vi "DAQmx Create Channel (TEDS-AI-Pressure-Bridge).vi"(0 "task in":refnum<k21>, 1 "maximum value":dbl=100.0 format="%0.2f", 2 "minimum value":dbl=-100.0 format="%0.2f", 5 "physical channels":tag, 7 "name to assign":string, 9 "units":i32(ring)=15879 items=["Pascals"=10081, "psi"=15879, "bar"=15880, "From Custom Scale"=10065], 11 "error in":errorcluster, 12 "custom scale name":tag, 13 "voltage excitation source":i32(ring)=10200 items=["Internal"=10200, "External"=10167], 14 "voltage excitation value":dbl=2.5) -> (4 "task out":refnum<k21>, 15 "error out":errorcluster)   [LabVIEW 2020]
doc: "Creates channel(s) that use a Wheatstone bridge to measure pressure. You must configure the physical channel(s) with TEDS information to use this VI. NI-DAQmx scales electrical values to physical values according to that TEDS information."
uses:
  nilvaiu.dll
panel:
  # "input limits"
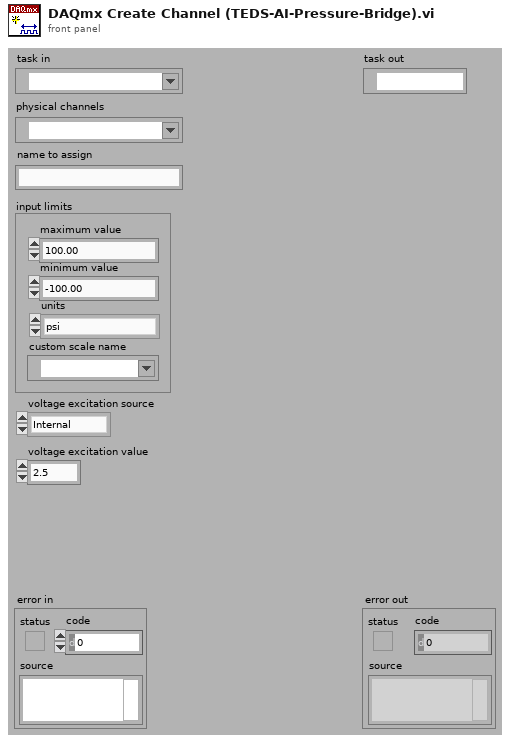
[diagram p1: front panel]
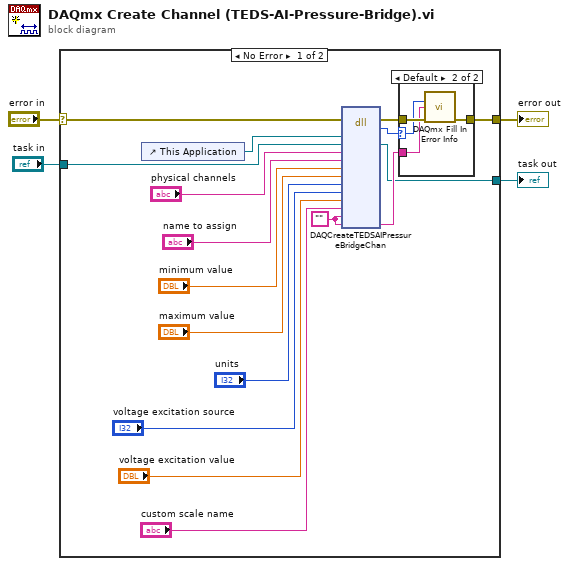
[diagram p0: block diagram]
diagram:
  n1 = case shown="No Error" "error in" {
    selector: "error in" -> [w11 w27]
    tunnel: [w18 w27] -> w4
    tunnel: "task in" -> [w14 w28]
    tunnel: [w17 w28] -> w1
    frame No Error {
      w5 = ""
      n2 = control-ref of="This Application"() -> (w16:refnum<vi>)
      n3 = dll-call lib="nilvaiu.*" fn="DAQCreateTEDSAIPressureBridgeChan"(error in=w11, "lvAppRef"=w16, "refObjPtr"=w14, "physicalChannelName"="physical channels", "channelNameIn"="name to assign", "minVal"="minimum value", "maxVal"="maximum value", "units"="units", "voltageExcitSource"="voltage excitation source", "voltageExcitVal"="voltage excitation value", "customScaleName"="custom scale name", "channelNamesOut"=w5, "extendedErrorInfo"=w5) -> (error out=w20:errorcluster, "return type"=w21:i32, "refObjPtr"=w17:refnum<k21>, "extendedErrorInfo"=w19:string)  [unwired: 12 in, 1 out]
      n4 = case shown="Default" w21 {
        selector: w21 -> [_ w24]
        tunnel: w20 -> [w22 w26]
        tunnel: [w22 w25] -> w18
        tunnel: w19 -> [_ w23]
        frame 0 {
        }
        frame Default {
          n5 = call "DAQmx Fill In Error Info.vi"("status code"=w24, "extended error info"=w23, "error in"=w26) -> ("error out"=w25:errorcluster)  [unwired: 1 in, 11 out]
        }
      }
    }
    frame Error {
    }
  }
  "error out" <- w4
  "task out" <- w1
